vi "New-ROIstuff.vi"(4 "exits position":T2, 5 "X Resolution":i32, 6 "rad scale":dbl, 7 "Y Resolution":i32, 9 "plat diam(cm)":dbl, 11 "ROI":T1) -> (2 "platform":T3, 3 "Array":bool[][](array[boolean]))   [LabVIEW 2019]
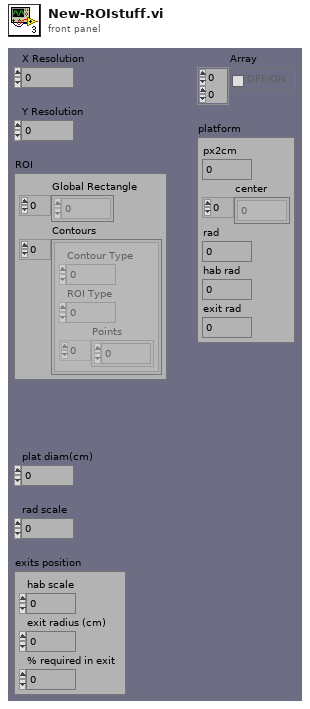
[diagram p1: front panel]
types:
  T1 = cluster{"Global Rectangle":i32[], "Contours":cluster{"Contour Type":u32, "ROI Type":u32, "Points":i32[]}[]}
  T2 = cluster{"hab scale":dbl, "exit radius (cm)":dbl, "% required in exit":dbl}
  T3 = cluster{"px2cm":dbl, "center":dbl[], "rad":dbl, "hab rad":dbl, "exit rad":dbl}
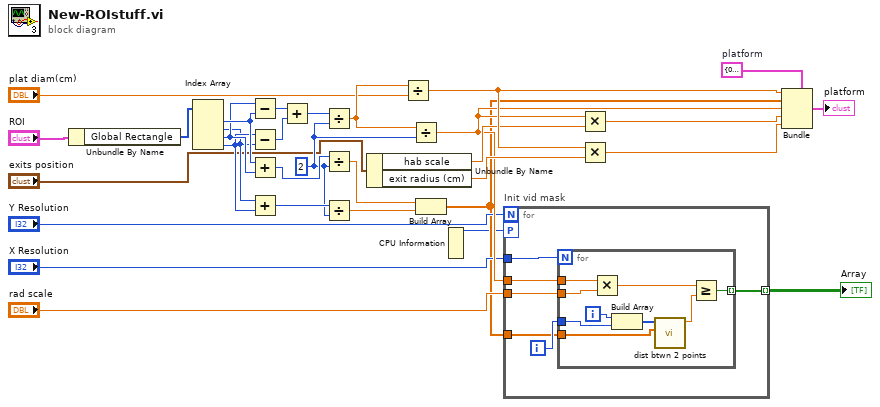
[diagram p0: block diagram]
diagram:
  w4 = T3 {"px2cm"=0.0, "center"=[0.0, 0.0], "rad"=0.0, "hab rad"=0.0, "exit rad"=0.0}  # platform
  w13 = 2
  n1 = Unbundle By Name("ROI") -> ("Global Rectangle"=w25:i32[])
  n2 = Index Array(array=w25) -> (element #1=w24:i32, element #2=w21:i32, element #3=w23:i32, element #4=w22:i32)  [unwired: 4 in]
  n3 = Subtract(x=w23, y=w24) -> (x-y=w18:i32)
  n4 = Subtract(x=w22, y=w21) -> (x-y=w17:i32)
  n5 = Add(x=w24, y=w23) -> (x+y=w20:i32)
  n6 = Add(x=w21, y=w22) -> (x+y=w19:i32)
  n7 = Add(x=w18, y=w17) -> (x+y=w16:i32)
  n8 = Divide(x=w16, y=w13) -> (x/y=w12:dbl)
  n9 = Divide(x=w20, y=w13) -> (x/y=w15:dbl)
  n10 = Divide(x=w19, y=w13) -> (x/y=w14:dbl)
  n11 = Unbundle By Name("exits position") -> ("hab scale"=w26:dbl, "exit radius (cm)"=w29:dbl)
  n12 = Divide(x=w12, y="plat diam(cm)") -> (x/y=w28:dbl)
  n13 = Divide(x=w12, y=w13) -> (x/y=w11:dbl)
  n14 = Build Array(w15, w14) -> (w5:dbl[])
  n15 = CPU Information() -> (4:w1:i32)  [unwired: 3 out]
  n16 = for "Init vid mask" {
    N: "Y Resolution" -> [_]
    tunnel: "X Resolution" -> [w37]
    tunnel: [w35] -> w7 mode=indexing
    tunnel: "rad scale" -> [w34]
    workers-P: w1 -> [_]
    tunnel: w11 -> [w33]
    tunnel: w5 -> [w32]
    i -> [w36]
    n17 = for {
      N: w37 -> [_]
      tunnel: w36 -> [w45]
      tunnel: [w43] -> w35 mode=indexing
      tunnel: w34 -> [w40]
      tunnel: w33 -> [w39]
      tunnel: w32 -> [w38]
      i -> [w46]
      n18 = Multiply(x=w39, y=w40) -> (x*y=w41:dbl)
      n19 = Build Array(w46, w45) -> (w44:i32[])
      n20 = call "dist btwn 2 points.vi"("coord pair 2"=w38, "coord pair1"=w44) -> ("dist"=w42:dbl)  [unwired: 9 in]
      n21 = Greater Or Equal?(x=w41, y=w42) -> (x >= y?=w43:bool)
    }
  }
  "Array" <- w7
  n22 = Multiply(x=w11, y=w26) -> (x*y=w27:dbl)
  n23 = Multiply(x=w28, y=w29) -> (x*y=w30:dbl)
  n24 = Bundle(cluster=w4, "px2cm"=w28, "center"=w5, "rad"=w11, "hab rad"=w27, "exit rad"=w30) -> (→"platform":T3)
